vi "NHRCapabilityTest.vi"() -> ()   [LabVIEW 2018]
uses:
  <instrlib>/niScope/Controls/niScope vertical coupling.ctl
  <vilib>/Utility/error.llb/DialogType.ctl
  <instrlib>/niScope/Acquire/Fetch/niScope Multi Fetch WDT.vi
  <instrlib>/NHRDCPowerModule/NHRDCPowerModule/NHRDCPowerModule.lvlib
panel:
  out "Stop NHR Collection?":bool
  out "Run Test?":bool
  out "Stop VI?":bool
  in  "NHR Disabled?":bool
  in  "Sample Rate":dbl=10000000.0 min=1.0 max=10000000.0 format="%_3p S/s"
  out "Scaled Current":waveform(dbl)(graph)
  out "Scaled Voltage":waveform(dbl)(graph)
  in  "Hold Time (ms)":sgl=100.0
  in  "Periods/Test":i32=10
  out "NHR On":bool
  in  "V/I Steps":i32=5
  out "Scope On":bool
  in  "Current vertical coupling":T1=1 items=["AC", "DC", "Ground"]
  in  "Current Channel Input Offset":dbl(ring) items=["+25"=25.0, "0"=0.0, "-25"=-25.0]
  out "Current Channel Range":dbl(ring)=10.0 items=["10A"=10.0, "35A"=35.0, "70A"=70.0]
  in  "Voltage vertical coupling":T1=1 items=["AC", "DC", "Ground"]
  in  "Voltage Channel Input Offset":dbl(ring) items=["+500"=500.0, "0"=0.0, "-500"=-500.0]
  out "Voltage Channel Range":dbl(ring)=700.0 items=["200V"=200.0, "700V"=700.0, "1400V"=1400.0]
  in  "Run Test":bool
  in  "Test":string(combo)="Voltage"
  in  "Stop VI":bool
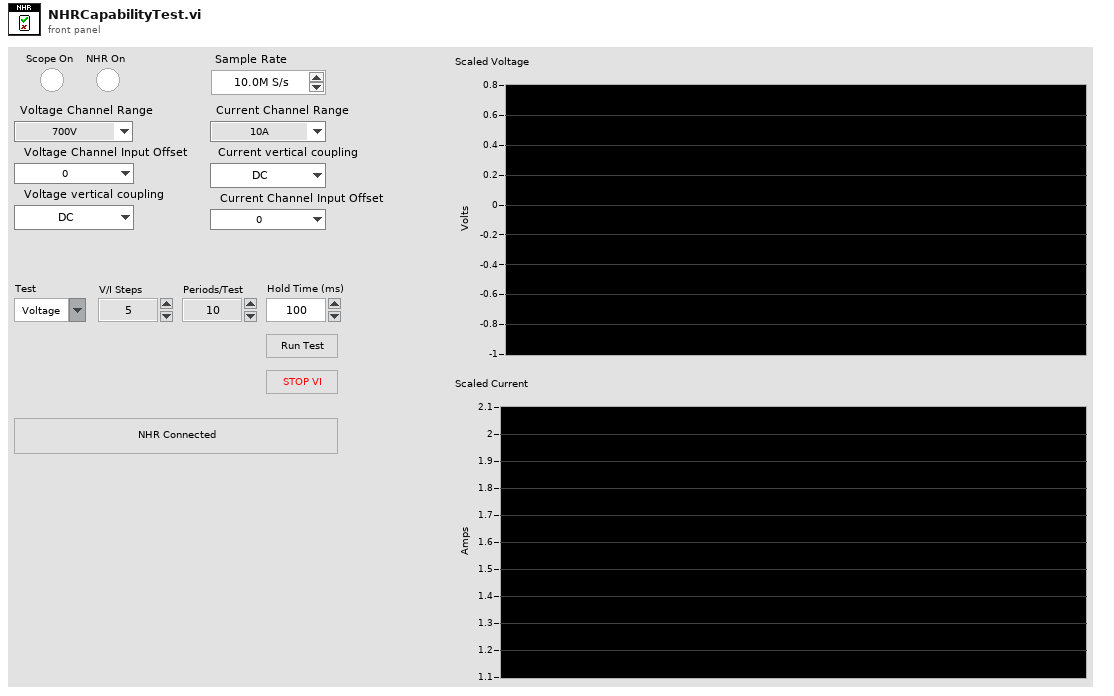
[diagram p1: front panel]
types:
  T1 = typedef "niScope vertical coupling.ctl" = i32
  T2 = enum16{"open", "open or create", "create or replace", "create", "open (read-only)"}
  T3 = typedef "DialogType.ctl" = u16
  T4 = typedef "LVStringsAndValuesArrayTypeDef_DBL.ctl" = cluster{"String":string, "Value":dbl}[]
  T5 = cluster{"actualSamples":i32, "absoluteInitialX":dbl, "relativeInitialX":dbl, "xIncrement":dbl, "offset":dbl, "gain":dbl, "reserved1":dbl, "reserved2":dbl}[]
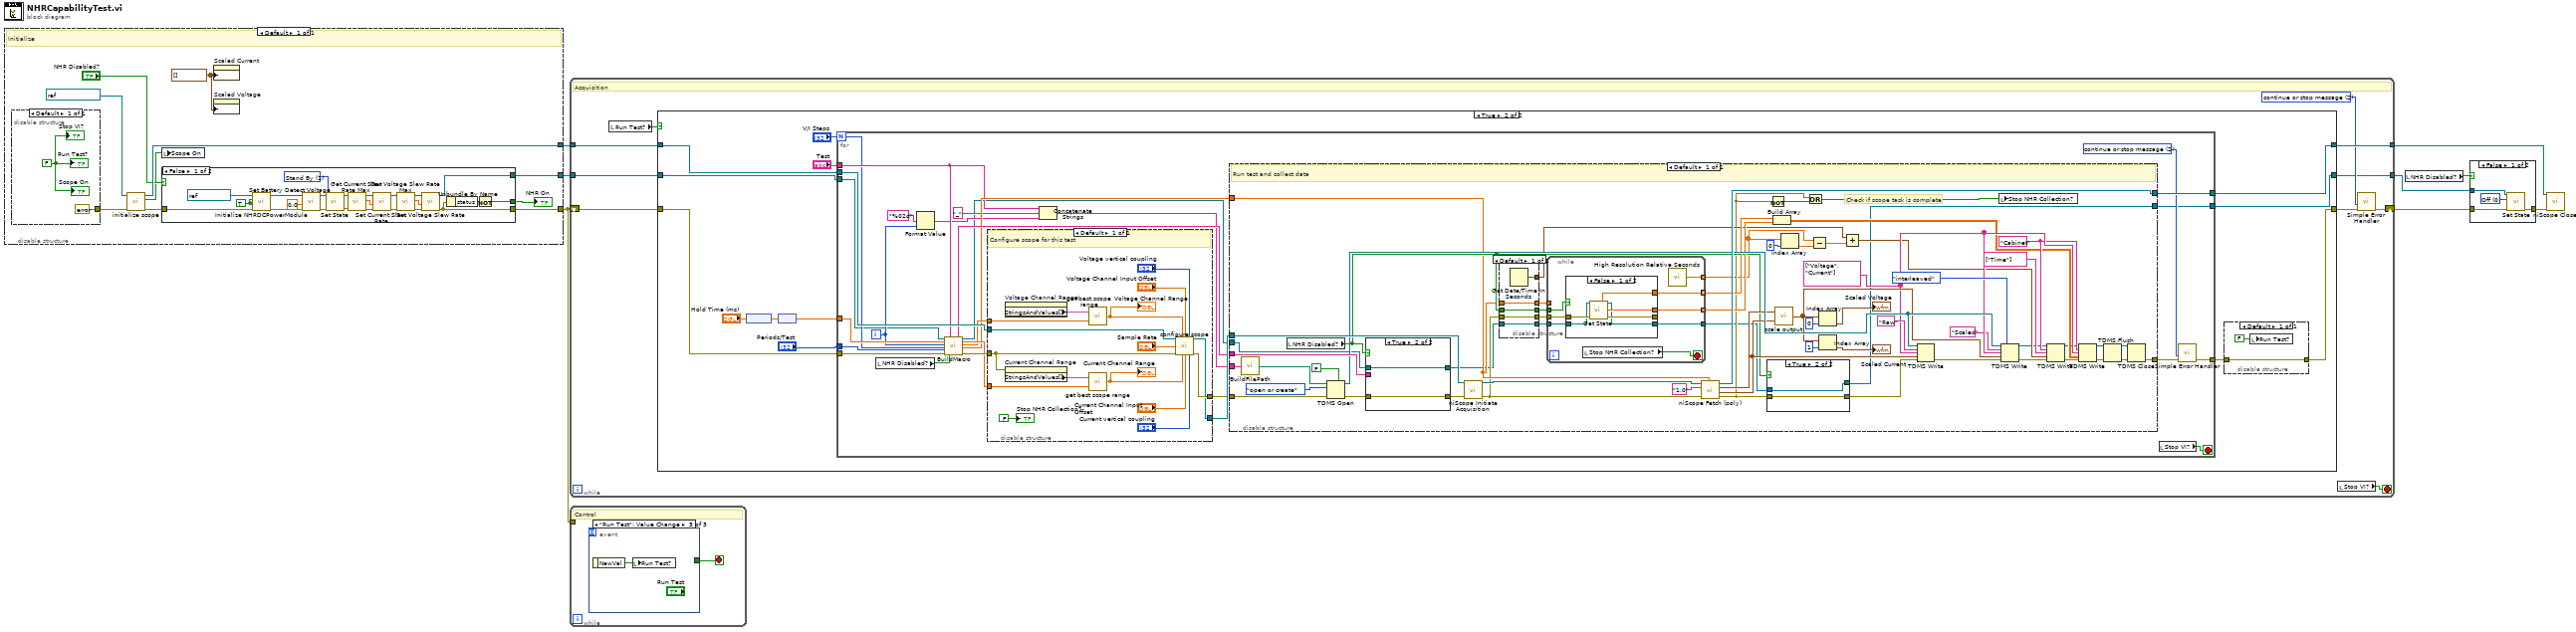
[diagram p0: block diagram]
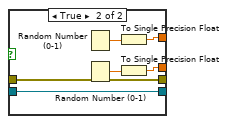
[diagram p3: hidden frame]
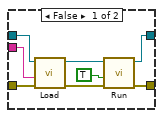
[diagram p4: hidden frame]
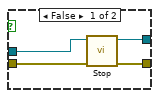
[diagram p5: hidden frame]
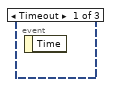
[diagram p6: hidden frame]
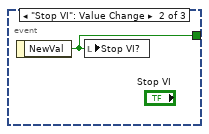
[diagram p7: hidden frame]
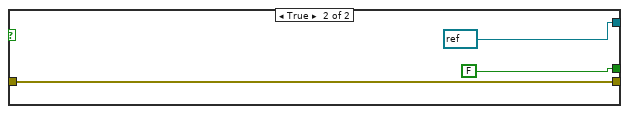
[diagram p9: hidden frame]
diagram:
  n1 = disable-structure shown="Default" {
    disable-tunnel: [w15] -> w8
    disable-tunnel: [w18] -> w7
    disable-tunnel: [w9] -> w1
    frame Enabled {
      w12 = waveform(dbl)[] [] ("History Data")
      # "Initialize"
      n2 = disable-structure shown="Default" {
        disable-tunnel: [errorcluster {"status"=FALSE, "code"=0, "source"=""} ("error in")] -> w11
        frame Enabled {
          w20 = FALSE ("Stop VI?")
          "Scope On" <- w20
          "Run Test?" <- w20
          "Stop VI?" <- w20
        }
      }
      n3 = call "initialize scope.vi"("error in"=w11, "resource name"=refnum<k15> "oscilloscope") -> ("error out"=w17:errorcluster, "Scope on"=w10:bool, "instrument handle"=w18:refnum<k15>)  [unwired: 2 in, 1 out]
      n4 = local write "Scope On"(w10) -> ()
      n5 = case shown="False" "NHR Disabled?" {
        tunnel: w17 -> [w43 w46]
        tunnel: [w42 w46] -> w15
        tunnel: [w21 FALSE ("status")] -> w14
        tunnel: [w30 refnum<visa-resource-name> refnum ("instrument handle out")] -> w9
        frame False {
          w22 = 1 items=["Off", "Stand By", "Charge", "Discharge", "Battery Emulation"] ("operating state (Off)")
          w40 = TRUE ("id query (Off)")
          n6 = call <instrlib>:"Initialize NHRDCPowerModule.vi"("error in (no error)"=w43, "reset device (Off)"=w40, "id query (Off)"=w40, "resource name"=refnum<visa-resource-name> "DC PM 1") -> ("error out"=w29:errorcluster, "instrument handle out"=w28:refnum<visa-resource-name>)  [unwired: 6 in]
          n7 = call <instrlib>:"Set Battery Detect Voltage.vi"("error in (no error)"=w29, "minimum voltage (4.0)"=sgl 0.0, "instrument handle"=w28) -> ("error out"=w25:errorcluster, "instrument handle out"=w26:refnum<visa-resource-name>)  [unwired: 7 in]
          n8 = call <instrlib>:"Set State.vi"("instrument handle"=w26, "operating state (Off)"=w22, "error in (no error)"=w25) -> ("instrument handle out"=w23:refnum<visa-resource-name>, "error out"=w24:errorcluster)  [unwired: 11 in]
          n9 = call <instrlib>:"Get Current Slew Rate Max.vi"("error in (no error)"=w24, "instrument handle"=w23) -> ("error out"=w38:errorcluster, "maximum current slew rate"=w39:sgl, "instrument handle out"=w37:refnum<visa-resource-name>)  [unwired: 7 in]
          n10 = call <instrlib>:"Set Current Slew Rate.vi"("error in (no error)"=w38, "current slew rate (0.0)"=w39, "instrument handle"=w37) -> ("error out"=w35:errorcluster, "instrument handle out"=w36:refnum<visa-resource-name>)  [unwired: 7 in]
          n11 = call <instrlib>:"Get Voltage Slew Rate Max.vi"("error in (no error)"=w35, "instrument handle"=w36) -> ("error out"=w32:errorcluster, "maximum voltage slew rate"=w33:sgl, "instrument handle out"=w34:refnum<visa-resource-name>)  [unwired: 7 in]
          n12 = call <instrlib>:"Set Voltage Slew Rate.vi"("error in (no error)"=w32, "voltage slew rate (0.0)"=w33, "instrument handle"=w34) -> ("error out"=w42:errorcluster, "instrument handle out"=w30:refnum<visa-resource-name>)  [unwired: 7 in]
          n13 = Unbundle By Name(w42) -> ("status"=w31:bool)
          n14 = Not(x=w31) -> (.not. x?=w21:bool)
        }
        frame True {
        }
      }
      "NHR On" <- w14
      n15 = property on="Scaled Current" class="WFChart (strict)"("History Data"=w12) -> ()  [unwired: 2 in, 2 out]
      n16 = property on="Scaled Voltage" class="WFChart (strict)"("History Data"=w12) -> ()  [unwired: 2 in, 2 out]
    }
  }
  n17 = while {
    shift-right: [w50] -> w6
    shift-left: w8 -> [w56]
    tunnel: w7 -> [w55]
    tunnel: [w54] -> w5
    tunnel: [w48] -> w2
    tunnel: w1 -> [w47]
    stop <- w51 stop-if-true
    w49 = T3 2 items=["no dialog", "OK message", "continue or stop message", "OK message + warnings", "continue/stop + warnings"] ("type of dialog (OK msg:1)")
    # "Acquisition"
    n18 = local read "Run Test?"() -> (w52:bool)
    n19 = case shown="True" w52 {
      tunnel: w56 -> [w58 w72]
      tunnel: w55 -> [w59 w71]
      tunnel: [w59 w70] -> w54
      tunnel: [w58 w64] -> w53
      tunnel: [w57 w61] -> w48
      tunnel: w47 -> [w57 w60]
      frame False {
      }
      frame True {
        n20 = node("Hold Time (ms)") -> (w63:sgl[unit])
        n21 = node(w63) -> (w62:sgl)
        n22 = for {
          N: "V/I Steps" -> [w82]
          tunnel: "Periods/Test" -> [w93]
          tunnel: "Test" -> [w84]
          tunnel: w62 -> [w94]
          tunnel: w72 -> [w96]
          tunnel: w71 -> [w99]
          tunnel: [w77] -> w65
          tunnel: [w97] -> w70
          tunnel: [w75] -> w61
          tunnel: w60 -> [w74]
          i -> [w80]
          stop <- w86 stop-if-true
          w76 = T3 2 items=["no dialog", "OK message", "continue or stop message", "OK message + warnings", "continue/stop + warnings"] ("type of dialog (OK msg:1)")
          n23 = local read "NHR Disabled?"() -> (w88:bool)
          n24 = Format Value(format string="%02d", value (0)=w80) -> (output string=w79:string)  [unwired: 1 in]
          n25 = call "BuildMacro.vi"("instrument handle"=w74, "Hold time (s)"=w94, "Current Test"=w80, "# Tests"=w82, "Periods/test"=w93, "error in"=w96, "Test type"=w84, "Enable NHR?"=w88) -> ("Macro file string"=w90:string, "instrument handle out"=w73:refnum<visa-resource-name>, "Max Current"=w92:dbl, "Max Voltage"=w91:dbl, "Test time"=w89:dbl, "error out"=w95:errorcluster)  [unwired: 6 in]
          n26 = disable-structure shown="Default" {
            disable-tunnel: w95 -> [w105]
            disable-tunnel: w99 -> [w115]
            disable-tunnel: w92 -> [w110]
            disable-tunnel: w91 -> [w109]
            disable-tunnel: [w103] -> w85
            disable-tunnel: [w102] -> w98
            frame Enabled {
              # "Configure scope for this test"
              n27 = property on="Voltage Channel Range" class="Ring (strict)"() -> ("StringsAndValues[]"=w107:T4)  [unwired: 2 in, 2 out]
              n28 = property on="Current Channel Range" class="Ring (strict)"(error in=w105) -> ("StringsAndValues[]"=w104:T4)  [unwired: 1 in, 2 out]
              n29 = call "get best scope range.vi"("Set point"=w109, "Range Strings and Values"=w107) -> ("Best Range"=w108:dbl)
              "Voltage Channel Range" <- w108
              n30 = call "get best scope range.vi"("Set point"=w110, "Range Strings and Values"=w104) -> ("Best Range"=w106:dbl)
              "Current Channel Range" <- w106
              n31 = call "configure scope.vi"("instrument handle"=w115, "Voltage Channel Range"=w108, "Voltage Channel Input Offset"="Voltage Channel Input Offset", "Voltage vertical coupling"="Voltage vertical coupling", "Sample Rate"="Sample Rate", "error in"=w105, "Current Channel Range"=w106, "Current Channel Input Offset"="Current Channel Input Offset", "Current vertical coupling"="Current vertical coupling") -> ("instrument handle out"=w102:refnum<k15>, "error out"=w103:errorcluster)  [unwired: 3 in, 2 out]
              "Stop NHR Collection?" <- FALSE
            }
          }
          n32 = Concatenate Strings(w84, "_" ("string"), w79) -> (w83:string)
          n33 = disable-structure shown="Default" {
            disable-tunnel: w90 -> [w175]
            disable-tunnel: w89 -> [w146]
            disable-tunnel: w98 -> [w172]
            disable-tunnel: [w170] -> w87
            disable-tunnel: [w169] -> w97
            disable-tunnel: w85 -> [w167]
            disable-tunnel: w83 -> [w154]
            disable-tunnel: [w117] -> w75
            disable-tunnel: w73 -> [w116]
            frame Enabled {
              w152 = "Cabinet" ("group name in (Untitled)")
              w153 = string[] ["Voltage", "Current"] ("channel name(s) in (Untitled)")
              # "Check if scope task is complete"
              # "Run test and collect data"
              n34 = call "BuildFilePath.vi"("File Name"=w154) -> ("Path"=w163:path)
              n35 = local read "NHR Disabled?"() -> (w147:bool)
              n36 = TDMS Open(5:FALSE ("create index file? (T)"), 8:w167, 10:T2."open or create" ("operation (0:open)"), 11:w163) -> (0:w166:errorcluster, 3:w165:refnum<k34>)  [unwired: 3 in]
              n37 = case shown="True" w147 {
                tunnel: w175 -> [w208 _]
                tunnel: [w207 w210] -> w142
                tunnel: w166 -> [w206 w210]
                tunnel: [w202 w209] -> w119
                tunnel: w116 -> [w201 w209]
                frame False {
                  n38 = call <instrlib>:"Load.vi"("error in (no error)"=w206, "path (\"\")"=w208, "instrument handle"=w201) -> ("error out"=w204:errorcluster, "instrument handle out"=w205:refnum<visa-resource-name>)  [unwired: 7 in]
                  n39 = call <instrlib>:"Run.vi"("error in (no error)"=w204, "continuous (false)"=TRUE, "instrument handle"=w205) -> ("error out"=w207:errorcluster, "instrument handle out"=w202:refnum<visa-resource-name>)  [unwired: 7 in]
                }
                frame True {
                }
              }
              n40 = call <instrlib>:"niScope Initiate Acquisition.vi"("instrument handle"=w172, "error in"=w142) -> ("instrument handle out"=w173:refnum<k15>, "error out"=w141:errorcluster)  [unwired: 12 in]
              n41 = disable-structure shown="Default" {
                disable-tunnel: w147 -> [w200]
                disable-tunnel: [w200] -> w134
                disable-tunnel: w146 -> [w199]
                disable-tunnel: [w199] -> w133
                disable-tunnel: w141 -> [w198]
                disable-tunnel: [w198] -> w132
                disable-tunnel: [w197] -> w145
                disable-tunnel: w119 -> [w196]
                disable-tunnel: [w196] -> w118
                frame Enabled {
                  n42 = Get Date/Time In Seconds() -> (seconds since 1Jan1904=w197:timestamp)
                }
              }
              n43 = while {
                tunnel: w132 -> [w183]
                tunnel: [w182] -> w149 mode=indexing
                tunnel: [w181] -> w150 mode=indexing
                tunnel: w134 -> [w180]
                tunnel: w133 -> [_]
                tunnel: [w179] -> w135 mode=indexing
                tunnel: w118 -> [w177]
                tunnel: [w176] -> w120
                stop <- w178 stop-if-true
                n44 = case shown="False" w180 {
                  tunnel: w183 -> [w189 w191]
                  tunnel: [w188 w193] -> w182
                  tunnel: [w187 w192] -> w181
                  tunnel: [w186 w191] -> _
                  tunnel: w177 -> [w185 w190]
                  tunnel: [w184 w190] -> w176
                  frame False {
                    n45 = call <instrlib>:"Get State.vi"("instrument handle"=w185, "error in (no error)"=w189) -> ("voltage"=w187:sgl, "instrument handle out"=w184:refnum<visa-resource-name>, "current"=w188:sgl, "error out"=w186:errorcluster)  [unwired: 3 in, 7 out]
                  }
                  frame True {
                    n46 = Random Number (0-1)() -> (number: 0 to 1=w194:dbl)
                    n47 = Random Number (0-1)() -> (number: 0 to 1=w195:dbl)
                    n48 = To Single Precision Float(number=w194) -> (single precision float=w192:sgl)
                    n49 = To Single Precision Float(number=w195) -> (single precision float=w193:sgl)
                  }
                }
                n50 = local read "Stop NHR Collection?"() -> (w178:bool)
                n51 = call <vilib>:"High Resolution Relative Seconds.vi"() -> ("relative seconds"=w179:dbl)
              }
              n52 = call-poly <instrlib>:"niScope Fetch (poly).vi"("timeout"=w146, "error in"=w141, "channels"="1,0", "instrument handle"=w173) -> ("error out"=w139:errorcluster, "wfm"=w161:waveform(dbl)[], "wfm info"=w162:T5, "instrument handle out"=w169:refnum<k15>)  [unwired: 4 in]
              n53 = case shown="True" w147 {
                tunnel: [w214 w216] -> w168
                tunnel: w139 -> [w213 w216]
                tunnel: w120 -> [w212 w215]
                tunnel: [w211 w215] -> w117
                frame False {
                  n54 = call <instrlib>:"Stop.vi"("error in (no error)"=w213, "instrument handle"=w212) -> ("error out"=w214:errorcluster, "instrument handle out"=w211:refnum<visa-resource-name>)  [unwired: 8 in]
                }
                frame True {
                }
              }
              n55 = Not(x=w139) -> (.not. x?=w140:bool)
              n56 = Build Array(w150, w149) -> (w148:sgl[][])
              n57 = call "scale output.vi"("Raw waveform"=w161, "wfm info"=w162) -> ("Scaled waveform"=w156:waveform(dbl)[])
              n58 = Index Array(array=w135, index=0) -> (element=w137:dbl)
              n59 = Or(x=w139, y=w140) -> (x .or. y?=w138:bool)
              n60 = Subtract(x=w135, y=w137) -> (x-y=w144:dbl[])
              n61 = Index Array(array=w156, index=0) -> (element=→"Scaled Voltage":waveform(dbl))
              n62 = Index Array(array=w156, index=1) -> (element=→"Scaled Current":waveform(dbl))
              n63 = Add(x=w145, y=w144) -> (x+y=w143:timestamp[])
              n64 = TDMS Write(0:w165, 5:"Raw" ("group name in (Untitled)"), 7:w153, 9:w161, 11:w168) -> (15:w128:errorcluster)  [unwired: 1 in, 3 out]
              n65 = local write "Stop NHR Collection?"(w138) -> ()
              n66 = TDMS Write(0:w165, 1:enum16{"decimated", "interleaved"}."interleaved" ("data layout (0:decimated)"), 5:"Scaled" ("group name in (Untitled)"), 7:w153, 9:w156, 11:w128) -> (4:w125:refnum<k34>, 15:w123:errorcluster)  [unwired: 2 out]
              n67 = TDMS Write(0:w125, 5:w152, 7:string[] ["Time"], 9:w143, 11:w123) -> (4:w124:refnum<k34>, 15:w122:errorcluster)  [unwired: 1 in, 2 out]
              n68 = TDMS Write(0:w124, 5:w152, 7:w153, 9:w148, 11:w122) -> (4:w126:refnum<k34>, 15:w127:errorcluster)  [unwired: 1 in, 2 out]
              n69 = TDMS Flush(4:w127, 7:w126) -> (0:w130:errorcluster, 3:w131:refnum<k34>)
              n70 = TDMS Close(8:w130, 11:w131) -> (0:w170:errorcluster)  [unwired: 1 out]
            }
          }
          n71 = local read "Stop VI?"() -> (w86:bool)
          n72 = call <vilib>:"Simple Error Handler.vi"("type of dialog (OK msg:1)"=w76, "error in (no error)"=w87) -> ("error out"=w77:errorcluster)  [unwired: 3 in, 4 out]
        }
        n73 = disable-structure shown="Default" {
          disable-tunnel: w65 -> [w217]
          disable-tunnel: [w217] -> w64
          frame Enabled {
            n74 = local write "Run Test?"(FALSE ("Run Test?")) -> ()
          }
        }
      }
    }
    n75 = local read "Stop VI?"() -> (w51:bool)
    n76 = call <vilib>:"Simple Error Handler.vi"("type of dialog (OK msg:1)"=w49, "error in (no error)"=w53) -> ("error out"=w50:errorcluster)  [unwired: 3 in, 4 out]
  }
  n77 = while {
    tunnel: w8 -> [_]
    stop <- w219 stop-if-true
    # "Control"
    n78 = event shown="[2] \"Run Test\": Value Change" {
      selector: _ -> [_ _ _]
      dyn-events: _ -> [_ _ _]
      timeout: _ -> [_ _ _]
      tunnel: [_ w220 _] -> w219
      event Timeout {
        n79 = event-data() -> ()  [unwired: 1 in, 1 out]
      }
      event "Stop VI": Value Change {
        n80 = event-data() -> ("NewVal"=w220:bool)  [unwired: 1 in]
        n81 = local write "Stop VI?"(w220) -> ()
      }
      event "Run Test": Value Change {
        n82 = event-data() -> ("NewVal"=w221:bool)  [unwired: 1 in]
        n83 = local write "Run Test?"(w221) -> ()
      }
    }
  }
  n84 = local read "NHR Disabled?"() -> (w3:bool)
  n85 = case shown="False" w3 {
    tunnel: w6 -> [w225 w226]
    tunnel: [w224 w226] -> w4
    tunnel: w2 -> [w222 _]
    frame False {
      w223 = 0 items=["Off", "Stand By", "Charge", "Discharge", "Battery Emulation"] ("operating state (Off)")
      n86 = call <instrlib>:"Set State.vi"("instrument handle"=w222, "operating state (Off)"=w223, "error in (no error)"=w225) -> ("error out"=w224:errorcluster)  [unwired: 11 in, 1 out]
    }
    frame True {
    }
  }
  n87 = call <instrlib>:"niScope Close.vi"("instrument handle"=w5, "error in"=w4) -> ()  [unwired: 13 in, 1 out]
